vi "Compute tau_phi & tau_m from Phasor (Discrete, Gated).vi"(8 "Error In":errorcluster, 9 "Phasor UCN[W] Parameters":T1, 10 "max tau":dbl[unit], 11 "Phasor":cluster{"X":dbl, "Y":dbl}) -> (0 "Error Out":errorcluster, 1 "Modulus Lifetime":dbl[unit], 3 "Phase Lifetime":dbl[unit], 5 "Modulus Lifetime Zeros":dbl[](array[numeric]) format="%.2f", 7 "Phase Lifetime Zeros":dbl[](array[numeric]) format="%.2f")   [LabVIEW 2019]
uses:
  Phasor UC_N[W] Parameters.ctl
  tau_phi & tau_m Zero Finder Parameters.ctl
  <vilib>/gmath/NI_Gmath.lvlib
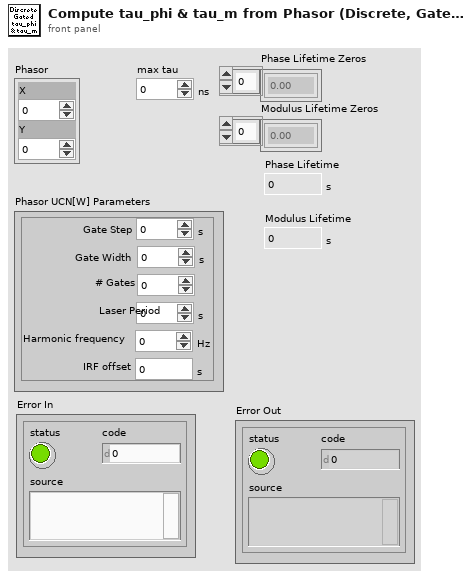
[diagram p1: front panel]
types:
  T1 = typedef "Phasor UC_N[W] Parameters.ctl" = cluster{"Laser Period":dbl[unit], "Gate Width":dbl[unit], "Gate Step":dbl[unit], "Harmonic frequency":dbl[unit], "IRF offset":dbl[unit], "# Gates":dbl}
  T2 = typedef "tau_phi & tau_m Zero Finder Parameters.ctl" = cluster{"Period":ext, "Width":ext, "# Gates":ext, "f":ext, "tan(phi), m":ext, "phi(T)/m(F)":bool, "Offset":ext}
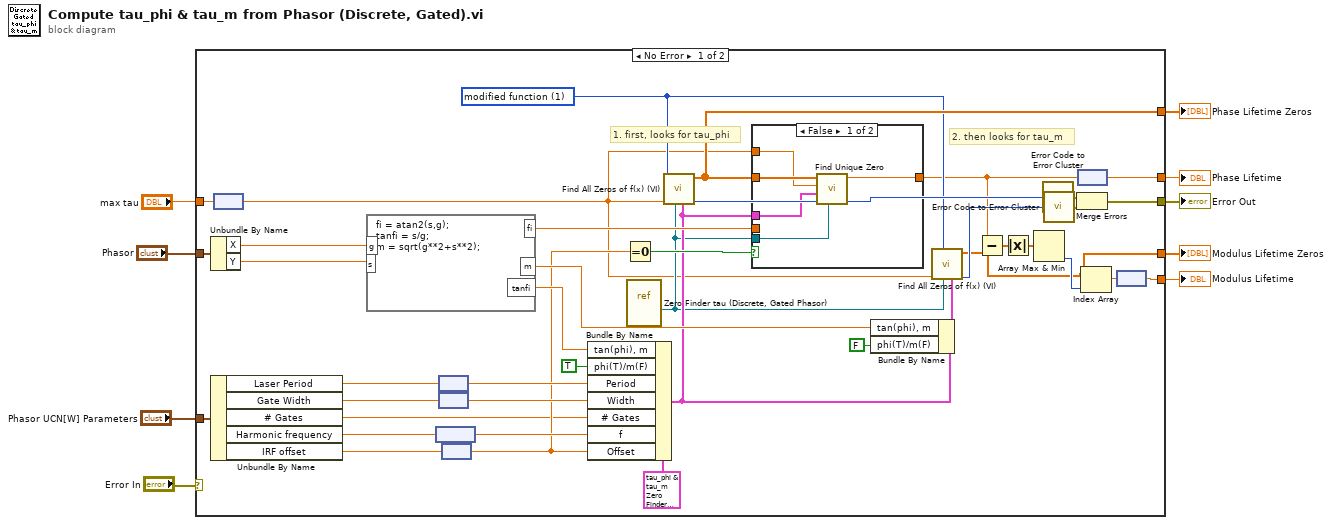
[diagram p0: block diagram]
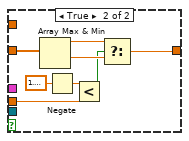
[diagram p2: hidden frame]
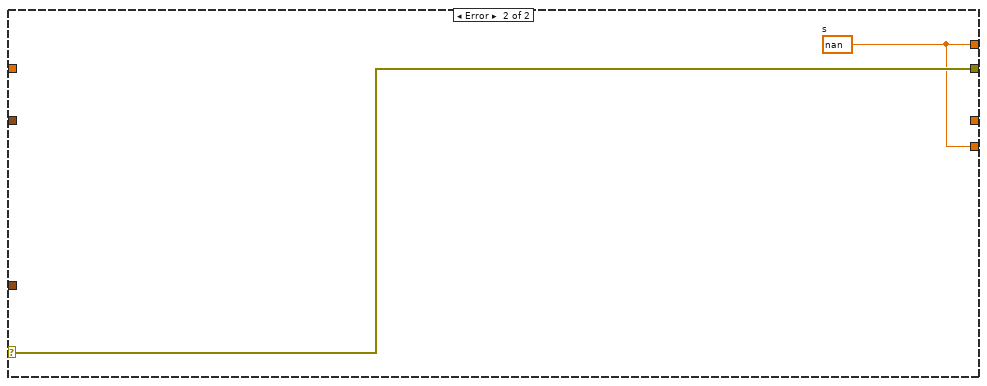
[diagram p3: hidden frame]
diagram:
  n1 = case shown="No Error" "Error In" {
    selector: "Error In" -> [_ w64]
    tunnel: "max tau" -> [w49 _]
    tunnel: [w48 _] -> w8
    tunnel: "Phasor" -> [w47 _]
    tunnel: [w38 w63] -> w6
    tunnel: [w32 w64] -> w5
    tunnel: [w30 w63] -> w4
    tunnel: [w25 _] -> w3
    tunnel: "Phasor UCN[W] Parameters" -> [w15 _]
    frame No Error {
      w31 = u16 1 items=["fixed function", "modified function"] ("step type")
      # "2. then looks for tau_m"
      # "1. first, looks for tau_phi"
      n2 = Unbundle By Name(w47) -> ("X"=w46:dbl, "Y"=w45:dbl)
      n3 = Unbundle By Name(w15) -> ("Laser Period"=w14:dbl[unit], "Gate Width"=w13:dbl[unit], "# Gates"=w10:dbl, "Harmonic frequency"=w12:dbl[unit], "IRF offset"=w11:dbl[unit])
      n4 = node(w49) -> (w16:dbl)
      n5 = formula code="fi = atan2(s,g);\ntanfi = s/g;\nm = sqrt(g**2+s**2);"("g"=w46, "s"=w45) -> ("tanfi"=w23:dbl, "m"=w39:dbl, "fi"=w20:dbl)
      n6 = node(w12) -> (w42:dbl)
      n7 = node(w14) -> (w44:dbl)
      n8 = node(w13) -> (w43:dbl)
      n9 = node(w11) -> (w21:dbl)
      n10 = Bundle By Name(cluster=T2 {"Period"=0.0, "Width"=0.0, "# Gates"=0.0, "f"=0.0, "tan(phi), m"=0.0, "phi(T)/m(F)"=TRUE, "Offset"=0.0}, "tan(phi), m"=w23, "phi(T)/m(F)"=TRUE, "Period"=w44, "Width"=w43, "# Gates"=w10, "f"=w42, "Offset"=w21) -> (w18:T2)
      n11 = Equal To 0?(x=w21) -> (x = 0?=w19:bool)
      n12 = vi-ref "Zero Finder tau (Discrete, Gated Phasor).vi"() -> (w17:refnum<vi>)
      n13 = call <vilib>:"Find All Zeros of f(x) (VI).vi"("data"=w18, "f(x)"=w17, "end"=w16, "step type"=w31) -> ("error"=w36:i32, "Zeros"=w48:dbl[])  [unwired: 4 in, 2 out]
      n14 = case shown="False" w19 {
        tunnel: w48 -> [w53 w62]
        tunnel: [w54 w59] -> w29
        tunnel: w20 -> [_ w58]
        tunnel: w18 -> [w51 _]
        tunnel: w17 -> [w50 _]
        tunnel: w16 -> [w52 _]
        frame False {
          n15 = call "Find Unique Zero.vi"("VI in"=w50, "Zero Finder Parameters"=w51, "max tau"=w52, "Zeros"=w53) -> ("Phase Lifetime"=w54:dbl)  [unwired: 6 in, 1 out]
        }
        frame True {
          n16 = Array Max & Min(array=w62) -> (max value=w61:dbl, min value=w60:dbl)  [unwired: 2 out]
          n17 = Negate(x=1.5707963267948966) -> (-x=w55:dbl)
          n18 = Less?(x=w55, y=w58) -> (x < y?=w57:bool)
          n19 = Select(t=w61, s=w57, f=w60) -> (s? t:f=w59:dbl)
        }
      }
      n20 = Bundle By Name(cluster=w18, "tan(phi), m"=w39, "phi(T)/m(F)"=FALSE) -> (w37:T2)
      n21 = call <vilib>:"Find All Zeros of f(x) (VI).vi"("data"=w37, "f(x)"=w17, "end"=w16, "step type"=w31) -> ("error"=w35:i32, "Zeros"=w25:dbl[])  [unwired: 4 in, 2 out]
      n22 = Subtract(x=w29, y=w25) -> (x-y=w28:dbl[])
      n23 = Absolute Value(x=w28) -> (abs(x)=w27:dbl[])
      n24 = Array Max & Min(array=w27) -> (min index (indices)=w26:i32)  [unwired: 3 out]
      n25 = call "Error Code to Error Cluster.vi"("Error Code"=w36) -> ("Error Out"=w34:errorcluster)
      n26 = call "Error Code to Error Cluster.vi"("Error Code"=w35) -> ("Error Out"=w33:errorcluster)
      n27 = Merge Errors(w34, w33) -> (w32:errorcluster)
      n28 = node(w29) -> (w30:dbl[unit])
      n29 = Index Array(array=w25, index=w26) -> (element=w24:dbl)
      n30 = node(w24) -> (w38:dbl[unit])
    }
    frame Error {
      w63 = dbl[unit] nan  # s
    }
  }
  "Modulus Lifetime" <- w6
  "Phase Lifetime" <- w4
  "Error Out" <- w5
  "Phase Lifetime Zeros" <- w8
  "Modulus Lifetime Zeros" <- w3
